vi "Scale.vi"(0 "From Min":dbl, 1 "From Max":dbl, 2 "Input Val":dbl, 3 "To Min":dbl, 4 "To Max":dbl) -> (5 "Output val":dbl, 6 "Integer Out":i64)   [LabVIEW 2015]
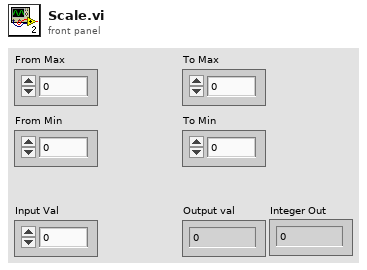
[diagram p1: front panel]
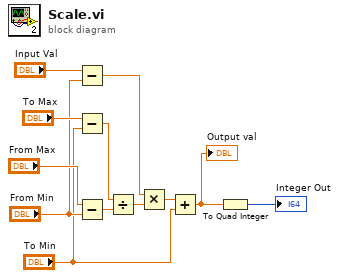
[diagram p0: block diagram]
diagram:
  n1 = Subtract(x="Input Val", y="From Min") -> (x-y=w5:dbl)
  n2 = Subtract(x="To Max", y="To Min") -> (x-y=w7:dbl)
  n3 = Subtract(x="From Max", y="From Min") -> (x-y=w6:dbl)
  n4 = Divide(x=w7, y=w6) -> (x/y=w4:dbl)
  n5 = Multiply(x=w5, y=w4) -> (x*y=w3:dbl)
  n6 = Add(x=w3, y="To Min") -> (x+y=w1:dbl)
  "Output val" <- w1
  n7 = To Quad Integer(1:w1) -> (0:→"Integer Out":i64)
